vi "MoveCamera.vi"(8 "error in (no error)":errorcluster, 10 "Refnum in":T5, 11 "TilesLoopData in":T1) -> (0 "error out":errorcluster, 3 "TilesLoopData out":T1)   [LabVIEW 2019, in "RT_Game.lvlib" / "Engine.lvclass"]
uses:
  Engine.lvclass
  TilesLoopData.ctl
  Game/Coordinate.ctl
  Game/SlideJob.ctl
  Game/ScreenSide.ctl
  FPGA_Interface.ctl
  <vilib>/Utility/error.llb/Error Cluster From Error Code.vi
  <vilib>/rvi/errors/niLvFpgaAdjustHostInterfaceError.vi
  <vilib>/rvi/interface/nirviReadWriteControl/nirviReadWriteControl.xnode
  FPGA Bitfiles/myriogameconsole_FPGATarget_Main_ntsPRcBZGxk.lvbitx
  NiFpgaLv.dll
  Game/Game.lvclass
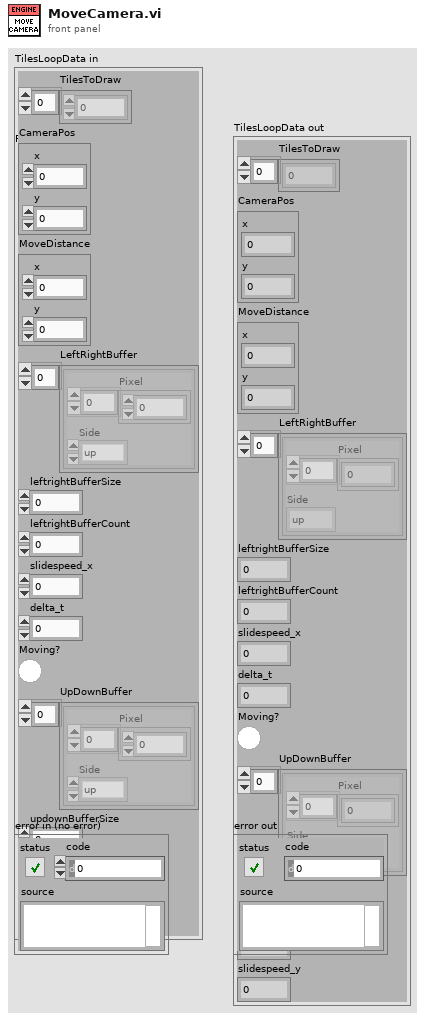
[diagram p1: front panel]
types:
  T1 = typedef "RT_Game.lvlib/Engine.lvclass/TilesLoopData.ctl" = cluster{"TilesToDraw":u64[], "CameraPos":T2, "MoveDistance":T2, "LeftRightBuffer":T3[], "leftrightBufferSize":i16, "leftrightBufferCount":i16, "slidespeed_x":dbl, "delta_t":dbl, "Moving?":bool, "UpDownBuffer":T3[], "updownBufferSize":i16, "updownBufferCount":i16, "slidespeed_y":dbl}
  T2 = typedef "RT_Game.lvlib/Game.lvclass/Coordinate.ctl" = cluster{"x":dbl, "y":dbl}
  T3 = typedef "RT_Game.lvlib/Engine.lvclass/SlideJob.ctl" = cluster{"Pixel":u32[], "Side":T4}
  T4 = typedef "RT_Game.lvlib/Game.lvclass/ScreenSide.ctl" = enum16{"up", "down", "left", "right", "none"}
  T5 = typedef "FPGA_Interface.ctl" = refnum<k20>
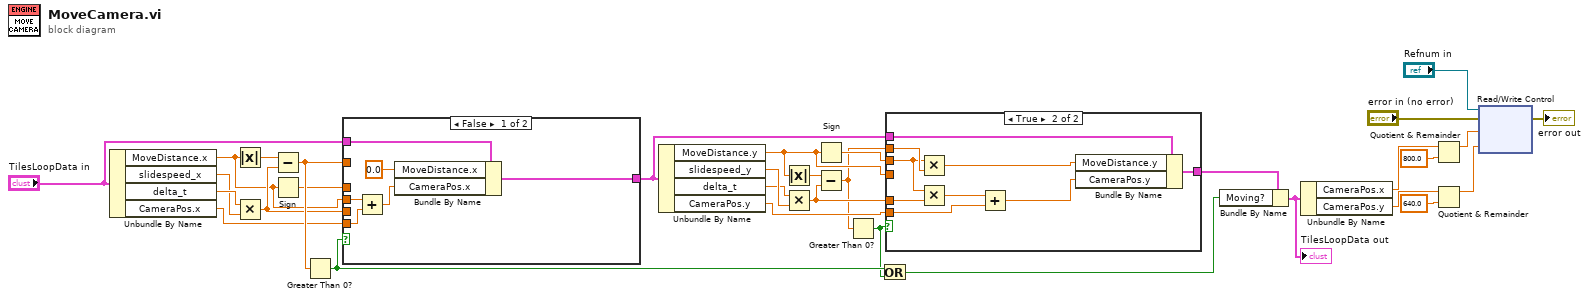
[diagram p0: block diagram]
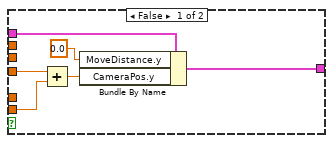
[diagram p2: hidden frame]
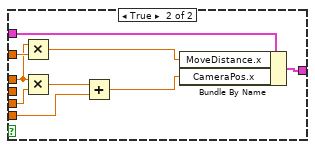
[diagram p3: hidden frame]
diagram:
  n1 = Unbundle By Name("TilesLoopData in") -> ("MoveDistance.x"=w16:dbl, "slidespeed_x"=w27:dbl, "delta_t"=w28:dbl, "CameraPos.x"=w23:dbl)
  n2 = Absolute Value(x=w16) -> (abs(x)=w26:dbl)
  n3 = Multiply(x=w28, y=w27) -> (x*y=w22:dbl)
  n4 = Subtract(x=w26, y=w22) -> (x-y=w30:dbl)
  n5 = Sign(1:w16) -> (0:w29:dbl)
  n6 = Greater Than 0?(x=w30) -> (x > 0?=w17:bool)
  n7 = case shown="False" w17 {
    tunnel: "TilesLoopData in" -> [w38 w47]
    tunnel: [w37 w46] -> w7
    tunnel: w29 -> [_ w39]
    tunnel: w30 -> [_ w44]
    tunnel: w23 -> [w35 w43]
    tunnel: w22 -> [_ w41]
    tunnel: w16 -> [w33 _]
    frame False {
      n8 = Add(x=w33, y=w35) -> (x+y=w34:dbl)
      n9 = Bundle By Name(cluster=w38, "MoveDistance.x"=0.0, "CameraPos.x"=w34) -> (w37:T1)
    }
    frame True {
      n10 = Multiply(x=w39, y=w44) -> (x*y=w45:dbl)
      n11 = Multiply(x=w39, y=w41) -> (x*y=w40:dbl)
      n12 = Add(x=w40, y=w43) -> (x+y=w42:dbl)
      n13 = Bundle By Name(cluster=w47, "MoveDistance.x"=w45, "CameraPos.x"=w42) -> (w46:T1)
    }
  }
  n14 = Unbundle By Name(w7) -> ("MoveDistance.y"=w15:dbl, "slidespeed_y"=w11:dbl, "delta_t"=w10:dbl, "CameraPos.y"=w13:dbl)
  n15 = Absolute Value(x=w15) -> (abs(x)=w12:dbl)
  n16 = Multiply(x=w10, y=w11) -> (x*y=w14:dbl)
  n17 = Sign(1:w15) -> (0:w9:dbl)
  n18 = Subtract(x=w12, y=w14) -> (x-y=w8:dbl)
  n19 = Greater Than 0?(x=w8) -> (x > 0?=w4:bool)
  n20 = Or(x=w17, y=w4) -> (x .or. y?=w5:bool)
  n21 = case shown="True" w4 {
    tunnel: w7 -> [w53 w62]
    tunnel: [w52 w61] -> w6
    tunnel: w9 -> [_ w54]
    tunnel: w8 -> [_ w59]
    tunnel: w13 -> [w50 w58]
    tunnel: w14 -> [_ w56]
    tunnel: w15 -> [w48 _]
    frame False {
      n22 = Add(x=w48, y=w50) -> (x+y=w49:dbl)
      n23 = Bundle By Name(cluster=w53, "MoveDistance.y"=0.0 ("MoveDistance.x"), "CameraPos.y"=w49) -> (w52:T1)
    }
    frame True {
      n24 = Multiply(x=w54, y=w59) -> (x*y=w60:dbl)
      n25 = Multiply(x=w54, y=w56) -> (x*y=w55:dbl)
      n26 = Add(x=w55, y=w58) -> (x+y=w57:dbl)
      n27 = Bundle By Name(cluster=w62, "MoveDistance.y"=w60, "CameraPos.y"=w57) -> (w61:T1)
    }
  }
  n28 = Bundle By Name(cluster=w6, "Moving?"=w5) -> (w18:T1)
  "TilesLoopData out" <- w18
  n29 = Unbundle By Name(w18) -> ("CameraPos.x"=w21:dbl, "CameraPos.y"=w2:dbl)
  n30 = Quotient & Remainder(x=w21, y=800.0 ("x")) -> (x-y*floor(x/y)=w19:dbl)  [unwired: 1 out]
  n31 = Quotient & Remainder(x=w2, y=640.0 ("x")) -> (x-y*floor(x/y)=w1:dbl)  [unwired: 1 out]
  n32 = xnode "Read/Write Control"("FPGA VI Reference In"="Refnum in", "error in"="error in (no error)", "x_Shift"=w19, "y_Shift"=w1) -> ("error out"=→"error out":errorcluster)  [unwired: 1 out]
